vi "Import File - Name Value Pair.vi"(6 "Root Node":refnum<k24>, 8 "error in (no error)":errorcluster, 11 "Node Name":string) -> (0 "error out":errorcluster, 4 "Value":string)   [LabVIEW 2019, in "UDP-Custom-Device System Explorer.lvlib"]
uses:
  UDP-Custom-Device System Explorer.lvlib
  System.Xml
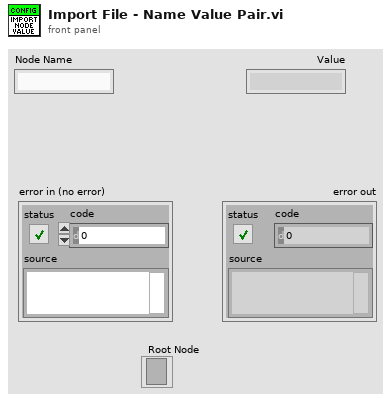
[diagram p1: front panel]
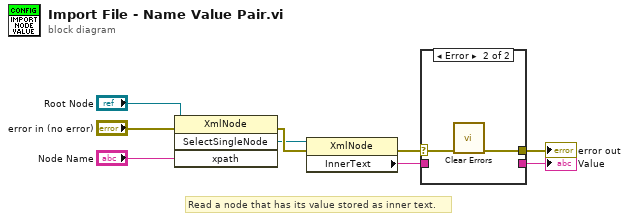
[diagram p0: block diagram]
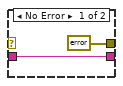
[diagram p2: hidden frame]
diagram:
  # "Read a node that has its value stored as inner text."
  n1 = invoke class="XmlNode" method="SelectSingleNode"(reference="Root Node", error in="error in (no error)", "xpath"="Node Name") -> (error out=w9:errorcluster, "SelectSingleNode"=w8:refnum<k24>)  [unwired: 1 in, 2 out]
  n2 = property class="XmlNode"(reference=w8, error in=w9) -> (error out=w2:errorcluster, "InnerText"=w3:string)  [unwired: 1 out]
  n3 = case shown="Error" w2 {
    selector: w2 -> [_ w13]
    tunnel: [w11 _] -> w4
    tunnel: w3 -> [w11 _]
    tunnel: [errorcluster {"status"=FALSE, "code"=0, "source"=""} ("error out") w12] -> w1
    frame No Error {
    }
    frame Error {
      n4 = call <vilib>:"Clear Errors.vi"("error in (no error)"=w13) -> ("error out"=w12:errorcluster)  [unwired: 5 in, 1 out]
    }
  }
  "error out" <- w1
  "Value" <- w4
